vi "test.assets_by_data_source.vi"() -> ()   [LabVIEW 2020]
uses:
  990e7071-dbe3-43dc-84d2-0d074c4f9026.vi
  Nominal Client/Nominal Client.lvclass
  asset/asset.lvclass
panel:
  out "Array":string[](array[string])
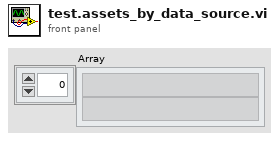
[diagram p1: front panel]
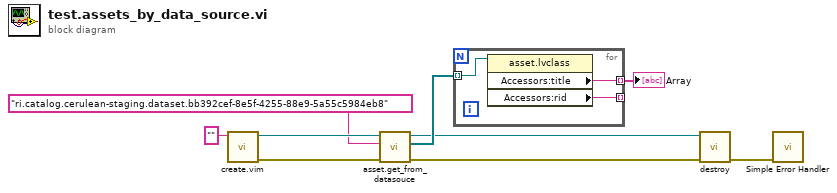
[diagram p0: block diagram]
diagram:
  n1 = call "create.vim"("API Token (string or path)"="") -> ("error out"=w6:errorcluster, "Nominal Client"=w7:refnum<class "Nominal Client.lvclass">)  [unwired: 9 in]
  n2 = call "asset.get_from_datasouce.vi"("error in"=w6, "Datasource RID"="ri.catalog.cerulean-staging.dataset.bb392cef-8e5f-4255-88e9-5a55c5984eb8", "Nominal Client in"=w7) -> ("error out"=w1:errorcluster, "Assets"=w3:refnum<class "asset.lvclass">[], "Nominal Client out"=w2:refnum<class "Nominal Client.lvclass">)  [unwired: 6 in]
  n3 = for {
    tunnel: w3 -> [w12] mode=indexing
    tunnel: [w11] -> _ mode=indexing
    tunnel: [w10] -> w4 mode=indexing
    n4 = property class="asset.lvclass"(reference=w12) -> ("Accessors:title"=w10:string, "Accessors:rid"=w11:string)  [unwired: 1 in, 2 out]
  }
  "Array" <- w4
  n5 = call "destroy.vi"("error in"=w1, "Nominal Client"=w2) -> ("error out"=w8:errorcluster)  [unwired: 9 in]
  n6 = call <vilib>:"Simple Error Handler.vi"("error in (no error)"=w8) -> ()  [unwired: 4 in, 5 out]
